vi "fgv_DO-daqmx.vi"(7 "cnt":T2, 8 "error in":errorcluster, 11 "Relay":cluster{"Relay":T1, "Boolean":bool}) -> (0 "error out":errorcluster)   [LabVIEW 2019]
uses:
  cnt_do.ctl
  cnt_Relay.ctl
  _ctrl/rw.ctl
  SubVIs/common/cmd_err.ctl
  <vilib>/DAQmx/write.llb/DAQmx Write (Digital 1D Bool NChan 1Samp 1Line).vi
  SubVIs/common/Glob_Ref.vi
  <vilib>/DAQmx/create/channels.llb/DAQmx Create Channel (DO-Digital Output).vi
  <vilib>/DAQmx/miscellaneous.llb/DAQmx Fill In Error Info.vi
  Durability/common/Global 1.vi
panel:
  out "data":bool[](array[boolean])
  out "Numeric":i32
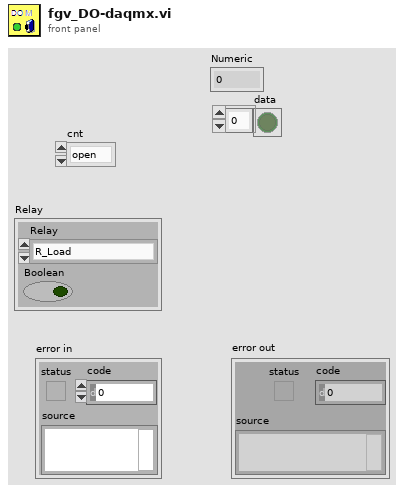
[diagram p1: front panel]
types:
  T1 = typedef "cnt_Relay.ctl" = enum32{"R_Load", "R_out1", "R_out2", "R_out3", "R_out4", "R_out5", "R_out6", "R8", "R9", "R10", "R11", "R12", "R13", "R14", "R15", "R16", "R_in1", "R_in2", "R_in3", "R_in4", "R_in5", "R_in6", "R23", "R24", "R25", "R26", "R27", "R_red", "R_yellow", "R_green", "R_buz", "R_purple"}
  T2 = typedef "cnt_do.ctl" = enum16{"open", "initial", "update", "run", "close"}
  T3 = enum16{"DL950", "BP4610", "DSP1500", "cDAQ-AI", "cDAQ-AO", "cDAQ-DO"}
  T4 = typedef "cmd_err.ctl" = enum16{"close", "open", "default"}
  T5 = typedef "rw.ctl" = enum16{"read", "write"}
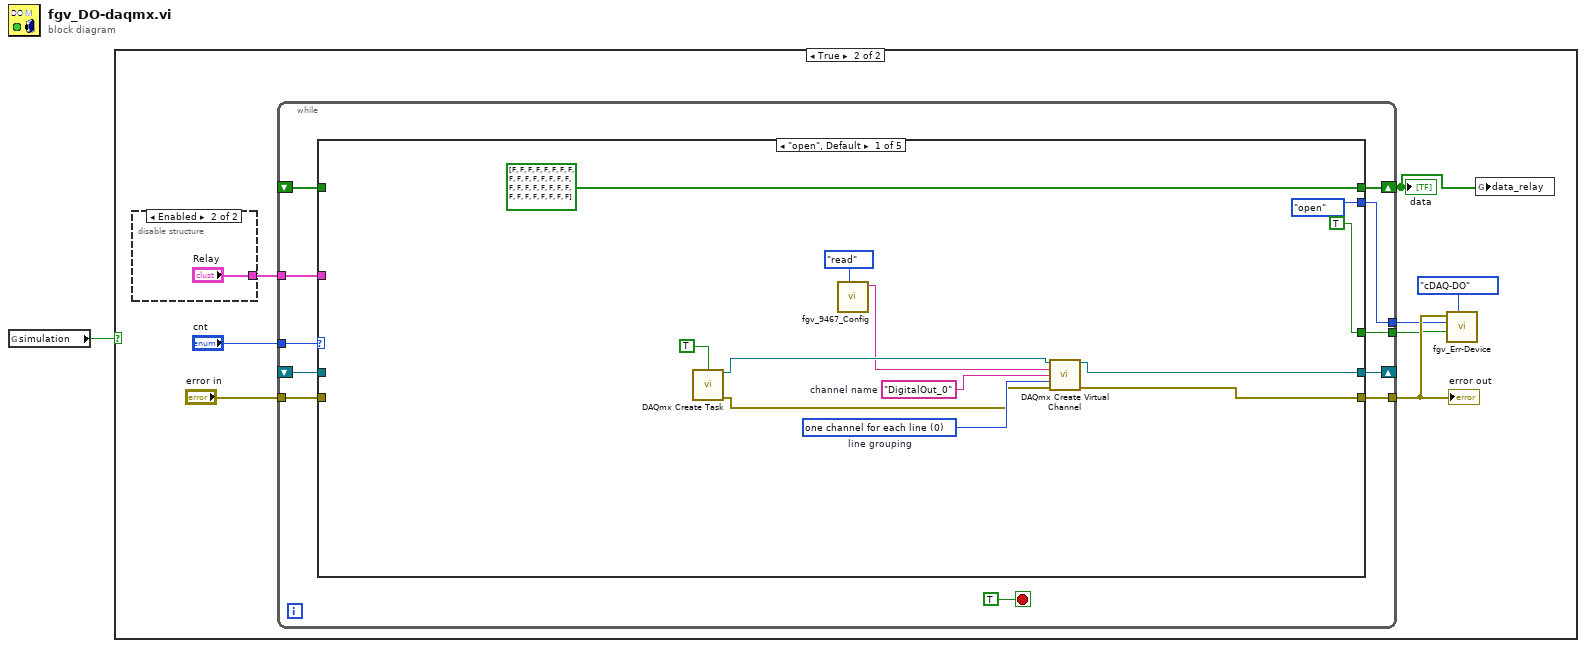
[diagram p0: block diagram]
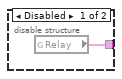
[diagram p3: hidden frame]
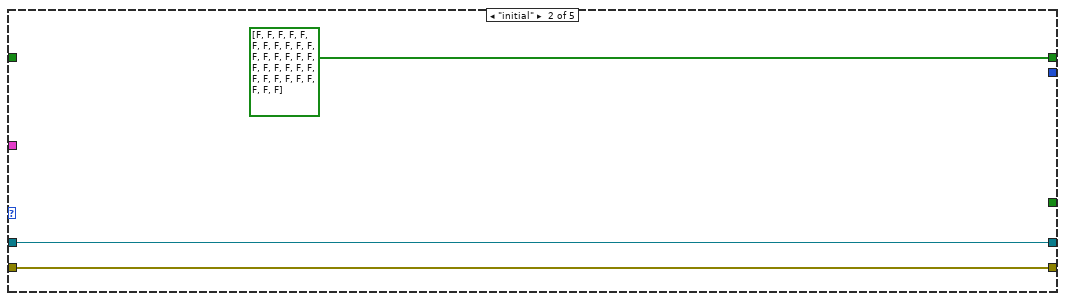
[diagram p4: hidden frame]
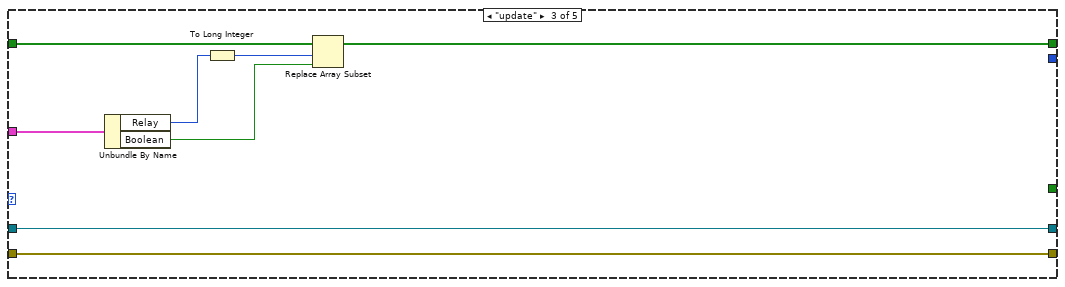
[diagram p5: hidden frame]
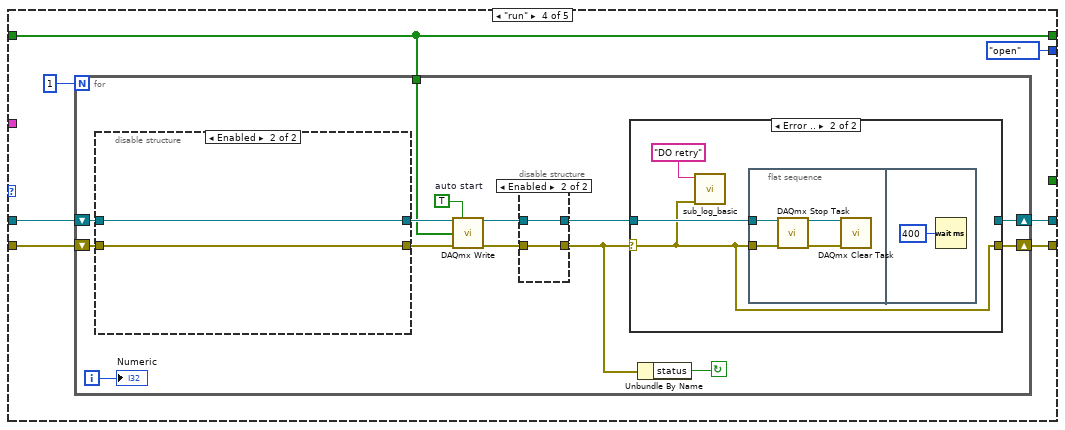
[diagram p6: hidden frame]
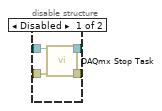
[diagram p7: hidden frame]
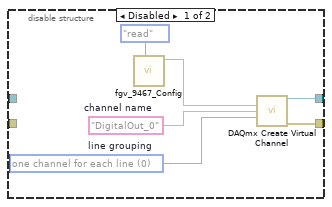
[diagram p8: hidden frame]
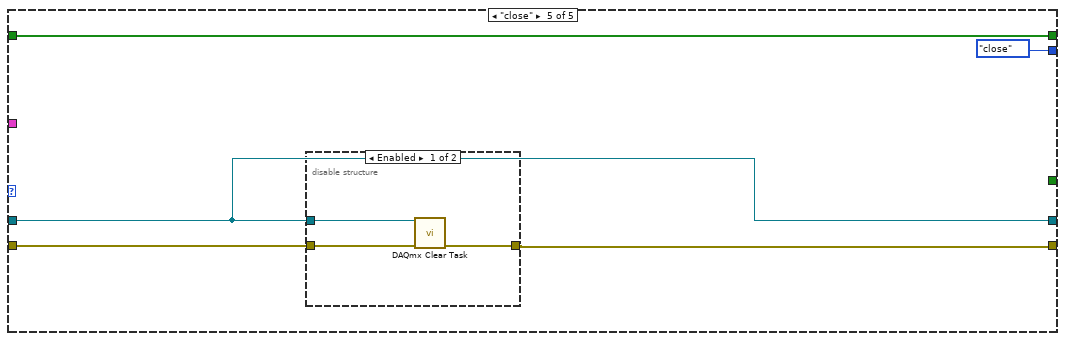
[diagram p10: hidden frame]
diagram:
  n1 = global read "Glob_Ref.vi" "simulation"() -> (w1:bool)
  n2 = case shown="True" w1 {
    frame False {
    }
    frame True {
      n3 = disable-structure shown="Enabled" {
        disable-tunnel: [w10 "Relay"] -> w5
        frame Disabled {
          n4 = global read "Global 1.vi" "Relay"() -> (w10:cluster{"Relay":T1, "Boolean":bool})
        }
        frame Enabled {
        }
      }
      n5 = while {
        tunnel: "cnt" -> [w21]
        shift-right: [w20] -> w2
        shift-left: _ -> [w19]
        tunnel: "error in" -> [w18]
        tunnel: [w17] -> w6
        tunnel: w5 -> [w16]
        shift-right: [w15] -> _
        shift-left: _ -> [w14]
        tunnel: [w13] -> w4
        tunnel: [w12] -> w3
        stop <- TRUE stop-if-true
        n6 = case shown="\"open\", Default" w21 {
          tunnel: [bool[] [FALSE, FALSE, FALSE, FALSE, FALSE, FALSE, FALSE, FALSE, FALSE, FALSE, FALSE, FALSE, FALSE, FALSE, FALSE, FALSE, FALSE, FALSE, FALSE, FALSE, FALSE, FALSE, FALSE, FALSE, FALSE, FALSE, FALSE, FALSE, FALSE, FALSE, FALSE, FALSE] ("data") bool[] [FALSE, FALSE, FALSE, FALSE, FALSE, FALSE, FALSE, FALSE, FALSE, FALSE, FALSE, FALSE, FALSE, FALSE, FALSE, FALSE, FALSE, FALSE, FALSE, FALSE, FALSE, FALSE, FALSE, FALSE, FALSE, FALSE, FALSE, FALSE, FALSE, FALSE, FALSE, FALSE] ("data") w44 w52 w95] -> w20
          tunnel: w19 -> [_ _ w45 w52 w95]
          tunnel: w18 -> [_ w36 w43 w48 w94]
          tunnel: [w26 w36 w43 w51 w92] -> w17
          tunnel: w16 -> [_ _ w41 _ _]
          tunnel: [w27 w35 w40 w50 w93] -> w15
          tunnel: w14 -> [_ w35 w40 w49 w93]
          tunnel: [cmd_err."open" ("cmd") _ _ cmd_err."open" ("cmd") cmd_err."close" ("cmd")] -> w13
          tunnel: [TRUE ("first?") _ _ _ _] -> w12
          frame "open", Default {
            w30 = 0 items=["one channel for each line", "one channel for all lines"]  # line grouping
            w31 = "DigitalOut_0"  # channel name
            n7 = call <vilib>:"DAQmx Create Task.vi"("auto cleanup"=TRUE) -> ("task out"=w29:refnum<k21>, "error out"=w25:errorcluster)  [unwired: 13 in]
            n8 = call "fgv_9467_Config.vi"("cmd"=rw."read") -> ("cDAQ-9467 Config 2"=w28:tag)  [unwired: 10 in]
            n9 = call-poly <vilib>:"DAQmx Create Virtual Channel.vi"("task in"=w29, "lines"=w28, "name to assign"=w31, "line grouping"=w30, "error in"=w25) -> ("task out"=w27:refnum<k21>, "error out"=w26:errorcluster)  [unwired: 9 in]
          }
          frame "initial" {
          }
          frame "update" {
            n10 = Unbundle By Name(w41) -> ("Relay"=w39:T1, "Boolean"=w38:bool)
            n11 = To Long Integer(number=w39) -> (32bit integer=w42:i32)
            n12 = Replace Array Subset(array=w45, new element=w38, index=w42) -> (w44:bool[])
          }
          frame "run" {
            n13 = for {
              N: 1 -> [_]
              tunnel: w52 -> [w60]
              shift-right: [w66] -> w51
              shift-left: w48 -> [w53]
              shift-right: [w65] -> w50
              shift-left: w49 -> [w54]
              i -> [w59]
              stop <- w64 continue-if-true
              w61 = TRUE  # auto start
              n14 = disable-structure shown="Enabled" {
                disable-tunnel: [w78 w79] -> w63
                disable-tunnel: [w77 w80] -> w62
                disable-tunnel: w54 -> [_ w80]
                disable-tunnel: w53 -> [_ w79]
                frame Disabled {
                  w75 = 0 items=["one channel for each line", "one channel for all lines"]  # line grouping
                  w76 = "DigitalOut_0"  # channel name
                  n15 = call "fgv_9467_Config.vi"("cmd"=rw."read") -> ("cDAQ-9467 Config 2"=w73:tag)  [unwired: 10 in]
                  n16 = call-poly <vilib>:"DAQmx Create Virtual Channel.vi"("lines"=w73, "name to assign"=w76, "line grouping"=w75) -> ("task out"=w77:refnum<k21>, "error out"=w78:errorcluster)  [unwired: 11 in]
                }
                frame Enabled {
                }
              }
              n17 = call-poly <vilib>:"DAQmx Write.vi"("task/channels in"=w62, "auto start"=w61, "data"=w60, "error in"=w63) -> ("task out"=w58:refnum<k21>, "error out"=w56:errorcluster)  [unwired: 9 in, 1 out]
              n18 = disable-structure shown="Enabled" {
                disable-tunnel: w58 -> [w70 w72]
                disable-tunnel: [w69 w72] -> w57
                disable-tunnel: w56 -> [w68 w71]
                disable-tunnel: [w67 w71] -> w55
                frame Disabled {
                  n19 = call <vilib>:"DAQmx Stop Task.vi"("task/channels in"=w70, "error in"=w68) -> ("task out"=w69:refnum<k21>, "error out"=w67:errorcluster)  [unwired: 12 in]
                }
                frame Enabled {
                }
              }
              n20 = case shown="Error .." w55 {
                selector: w55 -> [w82 w83]
                tunnel: [w82 w83] -> w66
                tunnel: [w81 _] -> w65
                tunnel: w57 -> [w81 w85]
                frame No Error {
                }
                frame Error {
                  n21 = call "sub_log_basic.vi"("error in"=w83, "Title"="DO retry") -> ()  [unwired: 9 in, 1 out]
                  n22 = flat-sequence {
                    tunnel: w85 -> [w89]
                    tunnel: w83 -> [w88]
                    frame #0 {
                      n23 = call <vilib>:"DAQmx Stop Task.vi"("task/channels in"=w89, "error in"=w88) -> ("task out"=w86:refnum<k21>, "error out"=w87:errorcluster)  [unwired: 12 in]
                      n24 = call <vilib>:"DAQmx Clear Task.vi"("task in"=w86, "error in"=w87) -> ()  [unwired: 13 in, 1 out]
                    }
                    frame #1 {
                      n25 = Wait (ms)(milliseconds to wait=u32 400) -> ()  [unwired: 1 out]
                    }
                  }
                }
              }
              n26 = Unbundle By Name(w55) -> ("status"=w64:bool)
              "Numeric" <- w59
            }
          }
          frame "close" {
            n27 = disable-structure shown="Enabled" {
              disable-tunnel: w94 -> [w97 _]
              disable-tunnel: w93 -> [w98 _]
              disable-tunnel: [w96 _] -> w92
              frame Enabled {
                n28 = call <vilib>:"DAQmx Clear Task.vi"("task in"=w98, "error in"=w97) -> ("error out"=w96:errorcluster)  [unwired: 13 in]
              }
              frame Disabled {
              }
            }
          }
        }
      }
      "error out" <- w6
      "data" <- w2
      n29 = call "fgv_Err-Device.vi"("Err Sel"=T3."cDAQ-DO", "first?"=w3, "cmd"=w4, "error in"=w6) -> ()  [unwired: 8 in]
      n30 = global write "Global 1.vi" "data_relay"(w2) -> ()
    }
  }
